vi "Write Traces.vi"(9 "New Data Queue":refnum<queue>, 10 "Traces":T1, 11 "User Interface in":refnum<class "User Interface.lvclass">) -> (3 "User Interface out":refnum<class "User Interface.lvclass">)   [LabVIEW 2016, in "User Interface.lvlib" / "User Interface.lvclass"]
uses:
  User Interface.lvclass
  Traces.ctl
  User Interface.lvclass/User Interface.ctl
  User Interface.lvlib
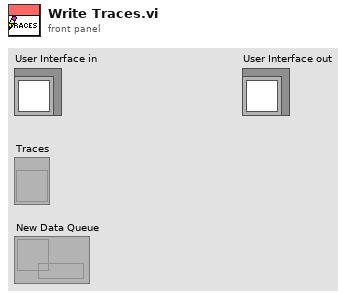
[diagram p1: front panel]
types:
  T1 = typedef "User Interface.lvlib/Traces.ctl" = refnum<vi>
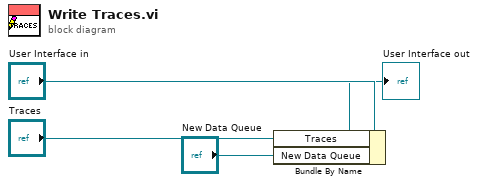
[diagram p0: block diagram]
diagram:
  n1 = Bundle By Name(cluster="User Interface in", "Traces"="Traces", "New Data Queue"="New Data Queue") -> (→"User Interface out":refnum<class "User Interface.lvclass">)
